vi "Verify Mock.vi"(8 "error in (no error)":errorcluster, 9 "Comparator":refnum<class "Comparator.lvclass">, 10 "Mock":refnum<class "Mock.lvclass">, 11 "LUnit Test Case In":refnum<class "Test Case.lvclass">) -> (0 "error out":errorcluster, 3 "LUnit Test Case Out":refnum<class "Test Case.lvclass">)   [LabVIEW 2020, in "Verifier.lvclass"]
uses:
  Verifier.lvclass
  <vilib>/Astemes/LUnit/Test Case.lvclass
  Mock/Mock.lvclass
  Comparator/Comparator.lvclass
  <vilib>/Astemes/LUnit/Test Case.lvclass/Test Case.ctl
  <vilib>/Astemes/LUnit/Append Fail Result.vi
  <vilib>/Astemes/LUnit/Append Pass Result.vi
  Verifier.lvclass/Verifier.ctl
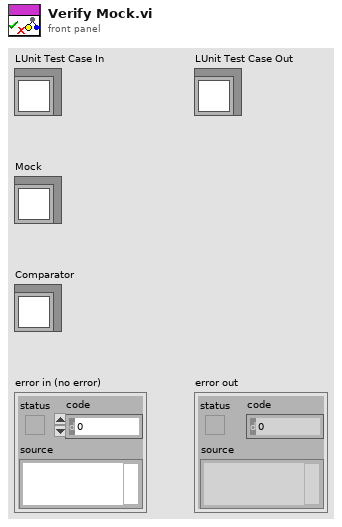
[diagram p1: front panel]
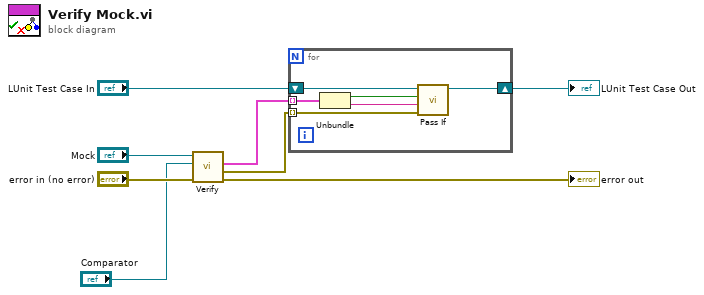
[diagram p0: block diagram]
diagram:
  n1 = call "Verify.vi"("error in (no error)"="error in (no error)", "Comparator"="Comparator", "Mock In"="Mock") -> ("error out"=→"error out":errorcluster, "Errors"=w3:errorcluster[], "Results"=w4:cluster{"Passed?":bool, "Message":string}[])  [unwired: 6 in]
  n2 = for {
    shift-right: [w13] -> w7
    shift-left: "LUnit Test Case In" -> [w14]
    tunnel: w4 -> [w11] mode=indexing
    tunnel: w3 -> [w12] mode=indexing
    n3 = Unbundle(w11) -> ("Passed?"=w10:bool, "Message"=w9:string)
    n4 = call <vilib>:"Pass If.vi"("error in (no error)"=w12, "Message"=w9, "Pass?"=w10, "LUnit Test Case In"=w14) -> ("LUnit Test Case Out"=w13:refnum<class "Test Case.lvclass">)  [unwired: 6 in, 1 out]
  }
  "LUnit Test Case Out" <- w7
